vi "MotorMultiInit.vi"(3 "Motors":string[](array[string]), 9 "error in (no error)":errorcluster) -> (0 "Motors out":string[](array[string]), 1 "Ok?":refnum<k4>[](array[refnum]), 6 "error out":errorcluster)   [LabVIEW 2009]
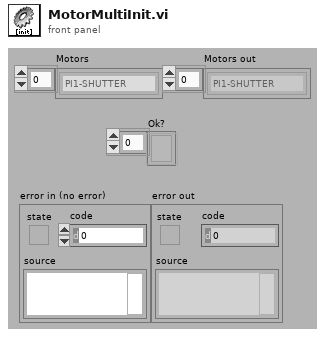
[diagram p1: front panel]
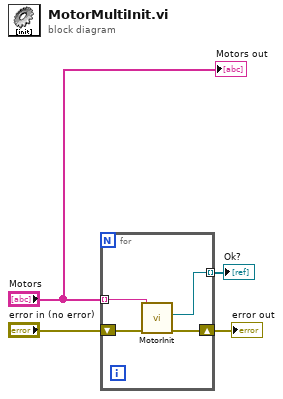
[diagram p0: block diagram]
diagram:
  n1 = for {
    tunnel: "Motors" -> [w6] mode=indexing
    shift-right: [w7] -> w3
    shift-left: "error in (no error)" -> [w8]
    tunnel: [w5] -> w1 mode=indexing
    n2 = call "MotorInit.vi"("Motor"=w6, "error in (no error)"=w8) -> ("Ok?"=w5:refnum<k4>, "error out"=w7:errorcluster)  [unwired: 6 out]
  }
  "error out" <- w3
  "Ok?" <- w1
  "Motors out" <- "Motors"
